vi "PQselect_Sample.vi"() -> ()   [LabVIEW 2019, in "libpqutility.lvlib"]
doc: "SELECT columns FROM table ---> Result Data\njust a sample"
uses:
  libpqutility.lvlib
  libpqlv/libpqlv.lvlib
panel:
  out "Data":string[][](table)
  out "PQresultStatus":T1(ring)
  out "PQresultErrorMessage":string
  out "PQerrorMessage":string
  out "PQStatus":T2(ring)
  in  "columns":string[](array[string])
  out "SELECTstring":string
  in  "table":string
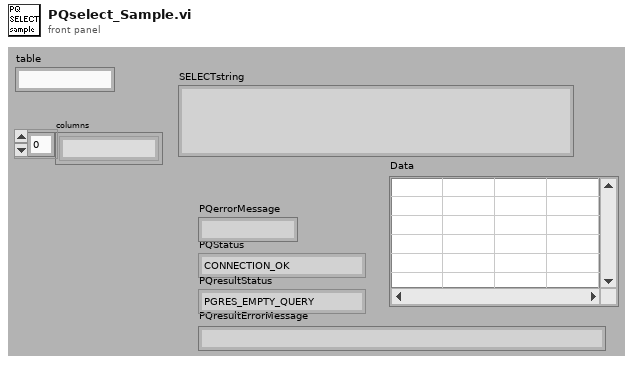
[diagram p1: front panel]
types:
  T1 = enum16{"PGRES_EMPTY_QUERY", "PGRES_COMMAND_OK", "PGRES_TUPLES_OK", "PGRES_COPY_OUT", "PGRES_COPY_IN", "PGRES_BAD_RESPONSE", "PGRES_NONFATAL_ERROR", "PGRES_FATAL_ERROR"}
  T2 = enum16{"CONNECTION_OK", "CONNECTION_BAD", "CONNECTION_STARTED", "CONNECTION_MADE", "CONNECTION_AWAITING_RESPONSE", "CONNECTION_AUTH_OK", "CONNECTION_SETENV", "CONNECTION_SSL_STARTUP", "CONNECTION_NEEDED"}
  T3 = enum32{"CONNECTION_OK", "CONNECTION_BAD", "CONNECTION_STARTED", "CONNECTION_MADE", "CONNECTION_AWAITING_RESPONSE", "CONNECTION_AUTH_OK", "CONNECTION_SETENV", "CONNECTION_SSL_STARTUP", "CONNECTION_NEEDED"}
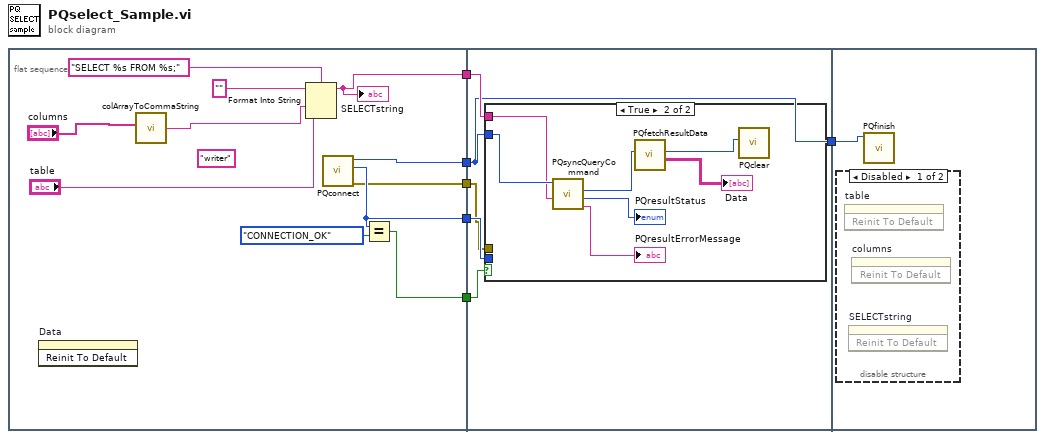
[diagram p0: block diagram]
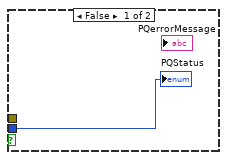
[diagram p2: hidden frame]
diagram:
  n1 = flat-sequence {
    tunnel: [w15] -> w6
    tunnel: [w14] -> w5
    tunnel: [w13] -> w4
    tunnel: [w12] -> w3
    tunnel: [w7] -> w1
    tunnel: w6 -> [w20]
    tunnel: w5 -> [w22]
    tunnel: w4 -> [w19]
    tunnel: w3 -> [w21]
    tunnel: [w19] -> w2
    tunnel: w1 -> [w18]
    tunnel: w2 -> [w31]
    frame #0 {
      (unwired) "writer" ("connection_name")
      n2 = invoke on="Data" class="Tbl (strikt)" method="Reinit To Default"() -> ()  [unwired: 3 in, 3 out]
      n3 = call "colArrayToCommaString.vi"("array"="columns") -> ("comma string"=w8:string)
      n4 = Format Into String(format string="SELECT %s FROM %s;" ("Format-String"), initial string="" ("Anfangsstring"), w8, "table") -> (resulting string=w12:string)  [unwired: 1 in, 1 out]
      "SELECTstring" <- w12
      n5 = call "PQconnect.vi"() -> ("error out"=w7:errorcluster, "PQStatus"=w14:T3, "conn"=w13:u32)  [unwired: 9 in]
      n6 = Equal?(x=w14, y=T2."CONNECTION_OK") -> (x = y?=w15:bool)
    }
    frame #1 {
      n7 = case shown="True" w20 {
        tunnel: w18 -> [_ _]
        tunnel: w22 -> [w23 _]
        tunnel: w19 -> [_ w30]
        tunnel: w21 -> [_ w29]
        frame False {
          "PQStatus" <- w23
        }
        frame True {
          n8 = call "PQsyncQueryCommand.vi"("query"=w29, "conn"=w30) -> ("PQresultErrorMessage"=→"PQresultErrorMessage":string, "PQresultStatus"=→"PQresultStatus":T1, "PGresult"=w26:u32)  [unwired: 5 in, 1 out]
          n9 = call "PQfetchResultData.vi"("res"=w26) -> ("Data"=→"Data":string[][], "res_out"=w25:u32)  [unwired: 5 in, 4 out]
          n10 = call "PQclear.vi"("res"=w25) -> ()  [unwired: 9 in, 2 out]
        }
      }
    }
    frame #2 {
      n11 = disable-structure shown="Disabled" {
        frame Disabled {
          n12 = invoke on="table" class="Str" method="Reinit To Default"() -> ()  [unwired: 3 in, 3 out]
          n13 = invoke on="SELECTstring" class="Str" method="Reinit To Default"() -> ()  [unwired: 3 in, 3 out]
          n14 = invoke on="columns" class="Arr (strikt)" method="Reinit To Default"() -> ()  [unwired: 3 in, 3 out]
        }
        frame Enabled {
        }
      }
      n15 = call "PQfinish.vi"("conn"=w31) -> ()  [unwired: 10 in, 1 out]
    }
  }
